vi "Hysteresis-CovarianceProcessing.vi"(11 "Covariances (2D)":dbl[][](array[numeric])) -> (2 "Covariance Processed (2D)":dbl[][](graph), 3 "Covariance Data":dbl[][](array[numeric]))   [LabVIEW 2016]
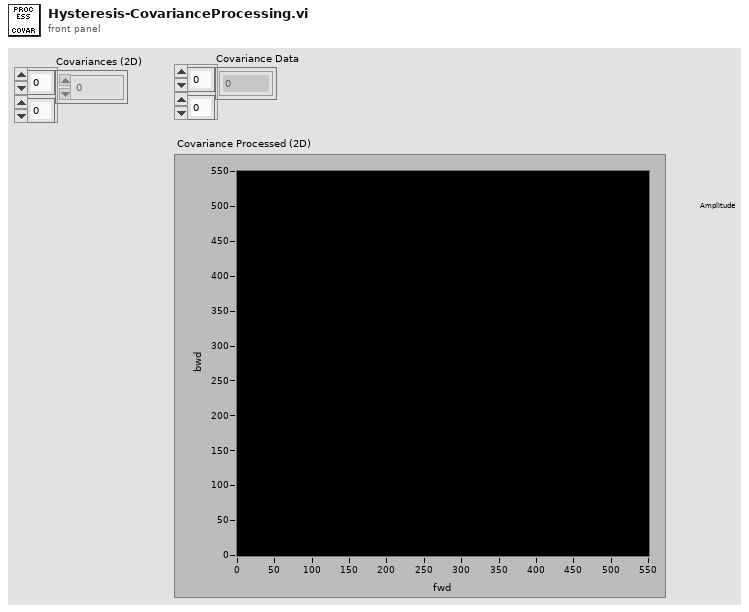
[diagram p1: front panel]
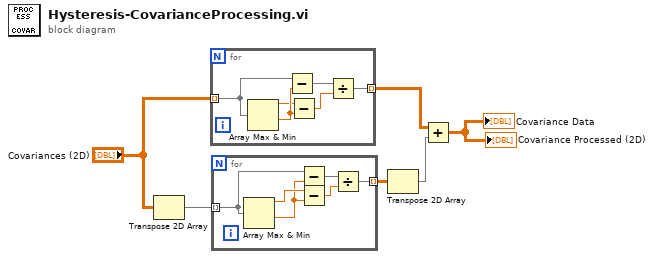
[diagram p0: block diagram]
diagram:
  n1 = Transpose 2D Array(2D array="Covariances (2D)") -> (transposed array=w2:dbl[][])
  n2 = for {
    tunnel: "Covariances (2D)" -> [w8] mode=indexing
    tunnel: [w7] -> w5 mode=indexing
    n3 = Array Max & Min(array=w8) -> (max value=w9:dbl, min value=w10:dbl)  [unwired: 2 out]
    n4 = Subtract(x=w8, y=w10) -> (x-y=w11:dbl[])
    n5 = Subtract(x=w9, y=w10) -> (x-y=w12:dbl)
    n6 = Divide(x=w11, y=w12) -> (x/y=w7:dbl[])
  }
  n7 = for {
    tunnel: w2 -> [w13] mode=indexing
    tunnel: [w14] -> w3 mode=indexing
    n8 = Array Max & Min(array=w13) -> (max value=w18:dbl, min value=w17:dbl)  [unwired: 2 out]
    n9 = Subtract(x=w13, y=w17) -> (x-y=w16:dbl[])
    n10 = Subtract(x=w18, y=w17) -> (x-y=w15:dbl)
    n11 = Divide(x=w16, y=w15) -> (x/y=w14:dbl[])
  }
  n12 = Transpose 2D Array(2D array=w3) -> (transposed array=w4:dbl[][])
  n13 = Add(x=w5, y=w4) -> (x+y=→"Covariance Processed (2D)" →"Covariance Data":dbl[][])
